vi "ErrorHandlerTest.vi"() -> ()   [LabVIEW 2019]
panel:
  in  "Power Cell":bool
  in  "Safties":bool
  in  "Tilt Interlock":bool
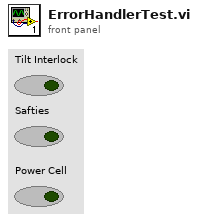
[diagram p1: front panel]
types:
  T1 = cluster{string, "Tilt Interlock":bool, "element":dbl}
  T2 = cluster{string, "Power Cell":bool, "element":dbl}
  T3 = cluster{string, "Power Cell":bool, "element":dbl}[]
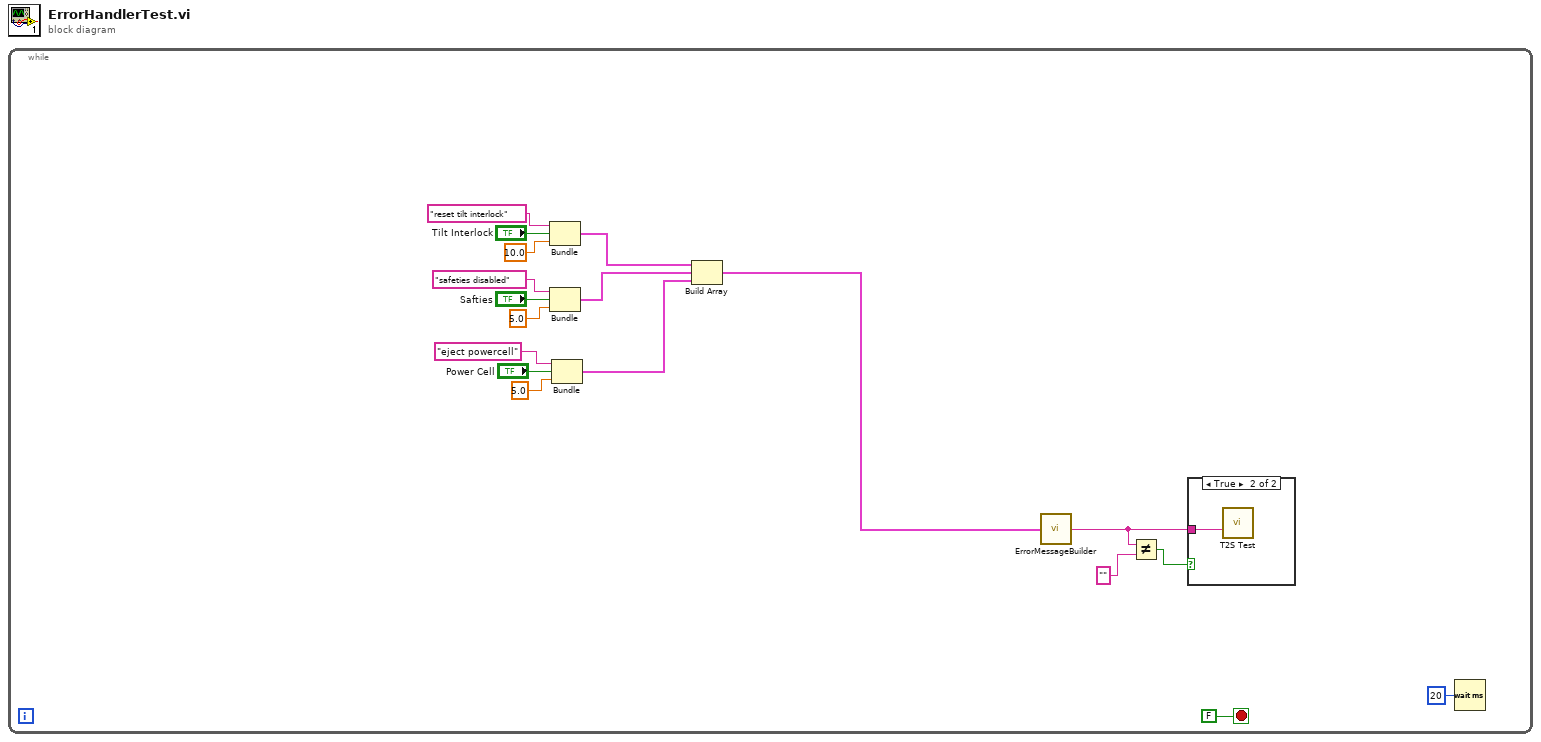
[diagram p0: block diagram]
diagram:
  n1 = while {
    stop <- FALSE stop-if-true
    n2 = Bundle("reset tilt interlock", "Tilt Interlock"="Tilt Interlock", "element"=10.0) -> (w13:T1)  [unwired: 1 in]
    n3 = Bundle("safeties disabled", "Safties"="Safties", "element"=5.0) -> (w9:cluster{string, "Safties":bool, "element":dbl})  [unwired: 1 in]
    n4 = Bundle("eject powercell", "Power Cell"="Power Cell", "element"=5.0) -> (w1:T2)  [unwired: 1 in]
    n5 = Build Array(w13, w9, w1) -> (w5:T3)
    n6 = call "ErrorMessageBuilder.vi"("Errors"=w5) -> ("Combined Error String"=w6:string)
    n7 = Not Equal?(x=w6, y="") -> (x != y?=w7:bool)
    n8 = case shown="True" w7 {
      tunnel: w6 -> [_ w19]
      frame False {
      }
      frame True {
        n9 = call "T2S Test.vi"("Text To Be Spoken"=w19) -> ()  [unwired: 9 in, 2 out]
      }
    }
    n10 = Wait (ms)(milliseconds to wait=u32 20) -> ()  [unwired: 1 out]
  }
